vi "Debounce Boolean.vi"(10 "cycles to filter (0)":u16, 11 "input":bool) -> (3 "filtered output":bool)   [LabVIEW 2017, in "NI_Robotics Utilities.lvlib"]
uses:
  <vilib>/robotics/Utilities/NI_Robotics Utilities.lvlib
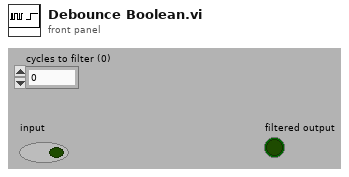
[diagram p1: front panel]
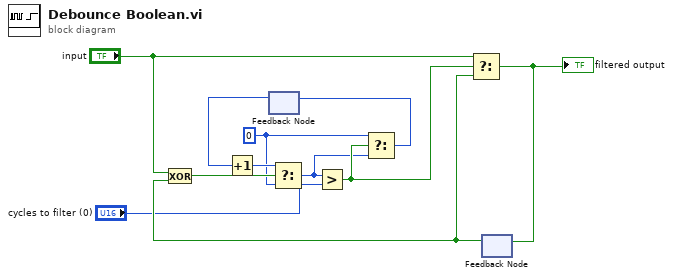
[diagram p0: block diagram]
diagram:
  w1 = u16 0 ("cycles to filter (0)")
  n1 = feedback #1() -> (w6:u16)  [unwired: 1 out]
  n2 = Increment(x=w6) -> (x+1=w5:u16)
  n3 = feedback #2() -> (w9:bool)  [unwired: 1 out]
  n4 = Exclusive Or(1:w9, 2:"input") -> (0:w8:bool)
  n5 = Select(t=w5, s=w8, f=w1) -> (s? t:f=w3:u16)
  n6 = Greater?(x=w3, y="cycles to filter (0)") -> (0:w4:bool)
  n7 = Select(t=w1, s=w4, f=w3) -> (s? t:f=w2:u16)
  n8 = feedback-in #1(w2) -> ()
  n9 = Select(t="input", s=w4, f=w9) -> (s? t:f=w10:bool)
  "filtered output" <- w10
  n10 = feedback-in #2(w10) -> ()
